vi "Treatment.vi"(8 "error in (no error)":errorcluster caption="entrée d'erreur (pas d'erreur)", 11 "Load_Wine en entrée":refnum<class "Load_Wine.lvclass">) -> (0 "error out":errorcluster caption="sortie d'erreur", 2 "Tableau":string[][](array[string]), 3 "Load_Wine en sortie":refnum<class "Load_Wine.lvclass">)   [LabVIEW 2020, in "Load_Wine.lvclass"]
uses:
  Load_Wine.lvclass
  Load_Wine.lvclass/Load_Wine.ctl
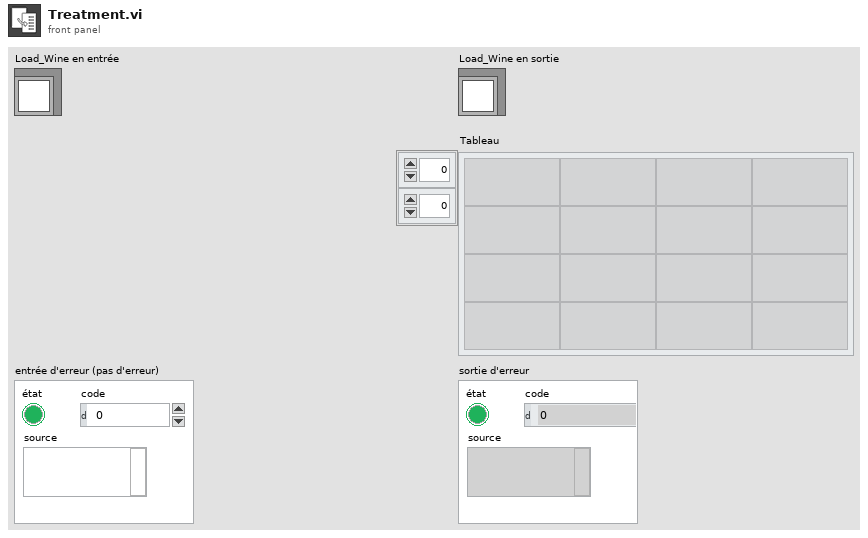
[diagram p1: front panel]
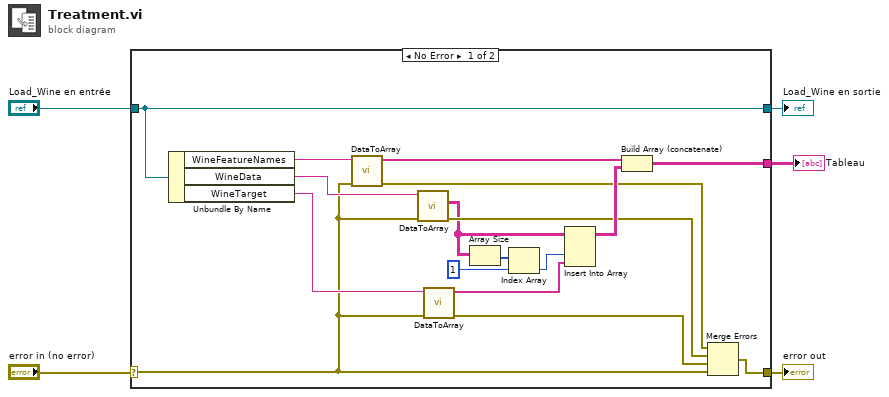
[diagram p0: block diagram]
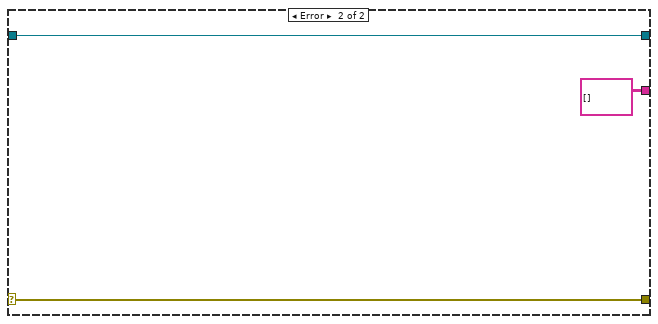
[diagram p2: hidden frame]
diagram:
  n1 = case shown="No Error" "error in (no error)" {
    selector: "error in (no error)" -> [w8 w25]
    tunnel: [w17 w25] -> w4
    tunnel: [w18 w24] -> w2
    tunnel: "Load_Wine en entrée" -> [w18 w24]
    tunnel: [w16 string[][] []] -> w1
    frame No Error {
      n2 = Unbundle By Name(w18) -> ("WineFeatureNames"=w15:string, "WineData"=w12:string, "WineTarget"=w9:string)
      n3 = call "DataToArray.vi"("sortie d'erreur"=w8, "Return value"=w15) -> ("sortie d'erreur"=w14:errorcluster, "String 1DArray"=w13:string[])  [unwired: 6 in, 2 out]
      n4 = call "DataToArray.vi"("sortie d'erreur"=w8, "Return value"=w12) -> ("sortie d'erreur"=w11:errorcluster, "String 2DArray"=w10:string[][])  [unwired: 6 in, 2 out]
      n5 = call "DataToArray.vi"("sortie d'erreur"=w8, "Return value"=w9) -> ("sortie d'erreur"=w6:errorcluster, "String 1DArray"=w7:string[])  [unwired: 6 in, 2 out]
      n6 = Array Size(array=w10) -> (size(s)=w21:i32[])
      n7 = Index Array(array=w21, index=1 ("indice")) -> (element=w20:i32)
      n8 = Insert Into Array(array=w10, index (col)=w20, new element=w7) -> (w22:string[][])  [unwired: 1 in]
      n9 = Build Array (concatenate)(w13, w22) -> (w16:string[][])
      n10 = Merge Errors(w14, w11, w6, w8) -> (w17:errorcluster)
    }
    frame Error {
    }
  }
  "error out" <- w4
  "Load_Wine en sortie" <- w2
  "Tableau" <- w1
